vi "5785_IQ_gen_2_x_1.6GHz_max_mod_8_and_4.vi"() -> ()   [LabVIEW 2021]
uses:
  <instrlib>/_niInstr/Streaming/v1/Common/Stream State.ctl
  <vilib>/Platform/TimedLoop/XDataNode/timing_clust.ctl
  <vilib>/Platform/TimedLoop/XDataNode/nitl_modes.ctl
  <vilib>/Platform/TimedLoop/XDataNode/wakeup.ctl
  <instrlib>/FlexRIO/API/FPGA/v1/Types/Start Trigger IO Resources.ctl
  <vilib>/rvi/Emulation/niFpgaSctlEmulationGetInTimedLoop.vi
  <vilib>/rvi/Emulation/niFpgaEmulationReportErrorSimple.vi
  <vilib>/rvi/Emulation/niFpgaGetClockAttributes.vi
  <vilib>/rvi/Emulation/niFpgaCriticalErrorInLSC.vi
  7192f61d-e408-4cca-baff-cb10c33219c0.vi
  <vilib>/rvi/interface/RandomDataEmulation/nirviRandomDataMultiElementFPGAFIFO.vi
  <instcachedir>/0/nirviRandomDataMultiElementFPGAFIFO_3E9965BA1FAD4E7B8DABA31768A09B1F.lvgen/nirviRandomDataMultiElementFPGAFIFO_3E9965BA1FAD4E7B8DABA31768A09B1F_000.vi
  <vilib>/rvi/interface/RandomDataEmulation/niFpgaRandomDataHandleErrors.vi
  <instrlib>/_niInstr/DSP/v1/FPGA/Public/Sub VIs/HB Interpolator/Halfband Interpolator - IQ - 8 SPC - 2x OC.vi
  <instrlib>/_niInstr/DSP/v1/FPGA/Public/Sub VIs/Frequency Shift/Frequency Shift - 16 spc.vi
  <vilib>/rvi/eio/common/nirviEmuTemplateMethod_errors.vi
  <vilib>/Platform/TimedLoop/XDataNode/XDataNode.xnode
  <vilib>/rvi/DataTransferAndStorage/Container/XNode/niFpgaContainer.xnode
  <vilib>/rvi/interface/RandomDataEmulation/nirviRandomDataFpgaMultiElementTemplate.vi
  <vilib>/eio/EIONode/EIONode.xnode
  <vilib>/Platform/TimedLoop/XDataNode/XDNodeRunTimeDep.lvlib
  <instrlib>/_niInstr/Streaming/v1/FPGA/niInstr Streaming v1 FPGA.lvlib
  <instrlib>/FlexRIO/API/FPGA/v1/FlexRIO API FPGA v1.lvlib
  <instrlib>/FlexRIO/API/FPGA/v1/IO/NI5785/FlexRIO 5785 FPGA v1.lvlib
  <instrlib>/_niInstr/DSP/v1/FPGA/niInstr DSP v1 FPGA.lvlib
  <instrlib>/_niInstr/Basic Elements/v1/FPGA/niInstr Basic Elements v1 FPGA.lvlib
  <instrlib>/_niInstr/Streaming/v1/Common/niInstr Streaming v1 Common.lvlib
panel:
  out "pulse TX status 2":T1
  out "pulse TX status":T1
  in  "reset system clock":bool
  in  "User-defined Start Trigger - AO":bool
  in  "flexrio.trigger.start.cfg 1":u16
  out "written elements":u64
  out "IO Socket\\AO Ready For Input":bool
  in  "stream.request state 1":T2
  in  "stream.num samples 1":u64
  out "stream.metadata 1":u64
  out "stream.samples transferred 1":u64
  out "stream.state 1":T2
  out "flexrio.module.io ready 0":bool
  out "flexrio.module.io error 0":i32
  out "flexrio.module.data valid 0":bool
  # "Data Path Configuration"
  # "AI Trigger Configuration"
  # "AI Stream Configuration"
  # "AO Stream Configuration"
  # "Module Status"
  # "AO Buffer Configuration"
  # "Device Utilization\n---------------------------\nTotal Slices: 62.6% (18977 out of 30300)\nSlice Registers: 23.8% (115206 out of 484800)\nSlice LUTs: 38.2% (92532 out of 242400)\nBlock RAMs: 56.8% (341 out of 600)\nDSP48s: 0.3% (6 out of 1920)\n\nNote: Utilization numbers are for the KU040. Exact values will vary for the KU060 and KU035."
  # "User-defined Controls"
  # "AO Trigger Configuration"
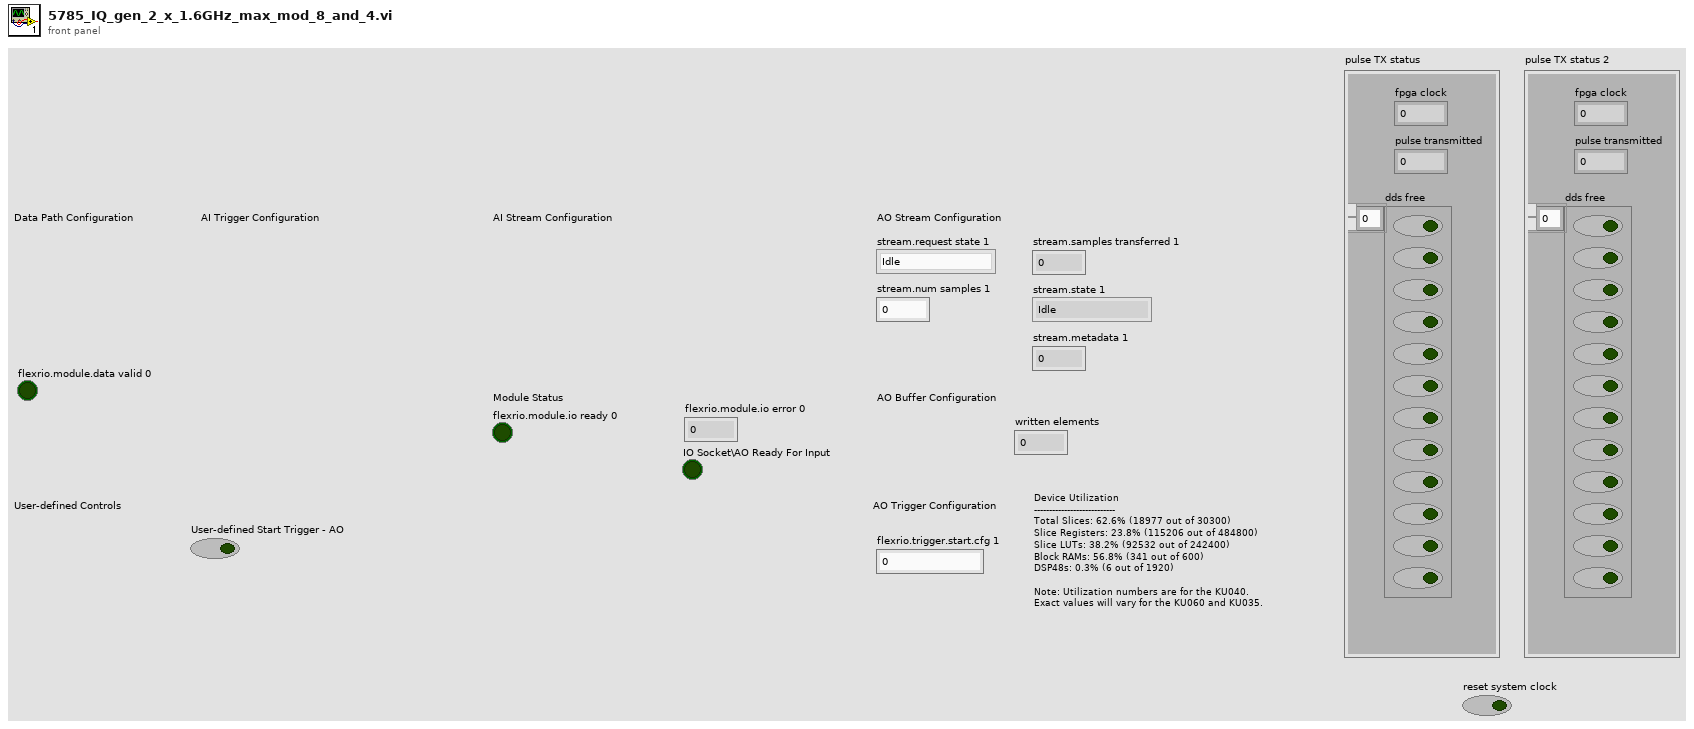
[diagram p1: front panel]
types:
  T1 = cluster{"fpga clock":u64, "pulse transmitted":u32, "dds free":bool[]}
  T2 = typedef "niInstr Streaming v1 Common.lvlib/Stream State.ctl" = enum8{"Idle", "Finite Transfer", "Continuous", "Done", "Error", "Not Ready", "Cancel"}
  T3 = typedef "XDNodeRunTimeDep.lvlib/timing_clust.ctl" = cluster{"Expected End [f-1]":u64, "Actual End [f-1]":u64, "Finished Late? [f-1]":bool, "Expected End [i-1]":u64, "Actual End [i-1]":u64, "Finished Late? [i-1]":bool, "Expected Start [i]":u64, "Actual Start [i]":u64, "Expected Start [f]":u64, "Actual Start [f]":u64, "Source Name":string, "Structure Name":string, "Period":i64, "Deadline":i64, "Offset":i64, "Start":i64, "Priority":i32, "Timeout":i32, "Mode":T4, "Wakeup Reason":T5, "Error":errorcluster, "Source Type":string, "Secondary Source Type":string, "Global End Time":u64, "Global Start Time":u64, "Frame Duration":u64, "Iteration Duration":u64, "Assigned CPU":i32, "I/O Scan Engine Mode":u32}
  T4 = typedef "XDNodeRunTimeDep.lvlib/nitl_modes.ctl" = enum32{"No Change", "Process missed periods, maintain original phase", "Discard missed periods, maintain original phase", "Process missed periods, ignore original phase", "Discard missed periods, ignore original phase"}
  T5 = typedef "XDNodeRunTimeDep.lvlib/wakeup.ctl" = enum32{"Normal", "Aborted", "Asynchronous wakeup", "Timing source error", "Timed loop error", "Timeout"}
  T6 = cluster{"Memory In":refnum<k21>, "Memory In 2":refnum<k21>, "Memory In 3":refnum<k21>, "Memory In 6":refnum<k21>, "Memory In 4":refnum<k21>, "Memory In 5":refnum<k21>, "Memory In 7":refnum<k21>, "Memory In 8":refnum<k21>}
  T7 = cluster{"clock x2":refnum<k21>, "Memory In":refnum<k21>, "Memory In 2":refnum<k21>, "Memory In 3":refnum<k21>, "Memory In 4":refnum<k21>}
  T8 = typedef "FlexRIO API FPGA v1.lvlib/Start Trigger IO Resources.ctl" = cluster{"start trigger":refnum<k21>, "started event":refnum<k21>, "start trigger for export":refnum<k21>, "start trigger for tclk":refnum<k21>}
  T9 = typedef "FlexRIO API FPGA v1.lvlib/Start Trigger Control.ctl" = cluster{"arm start":bool, "done":bool}
  T10 = typedef "niInstr DSP v1 Shared.lvlib/IQ Data.ctl" = cluster{"I":fxp<+/-,18,1>, "Q":fxp<+/-,18,1>, "overflow":bool}
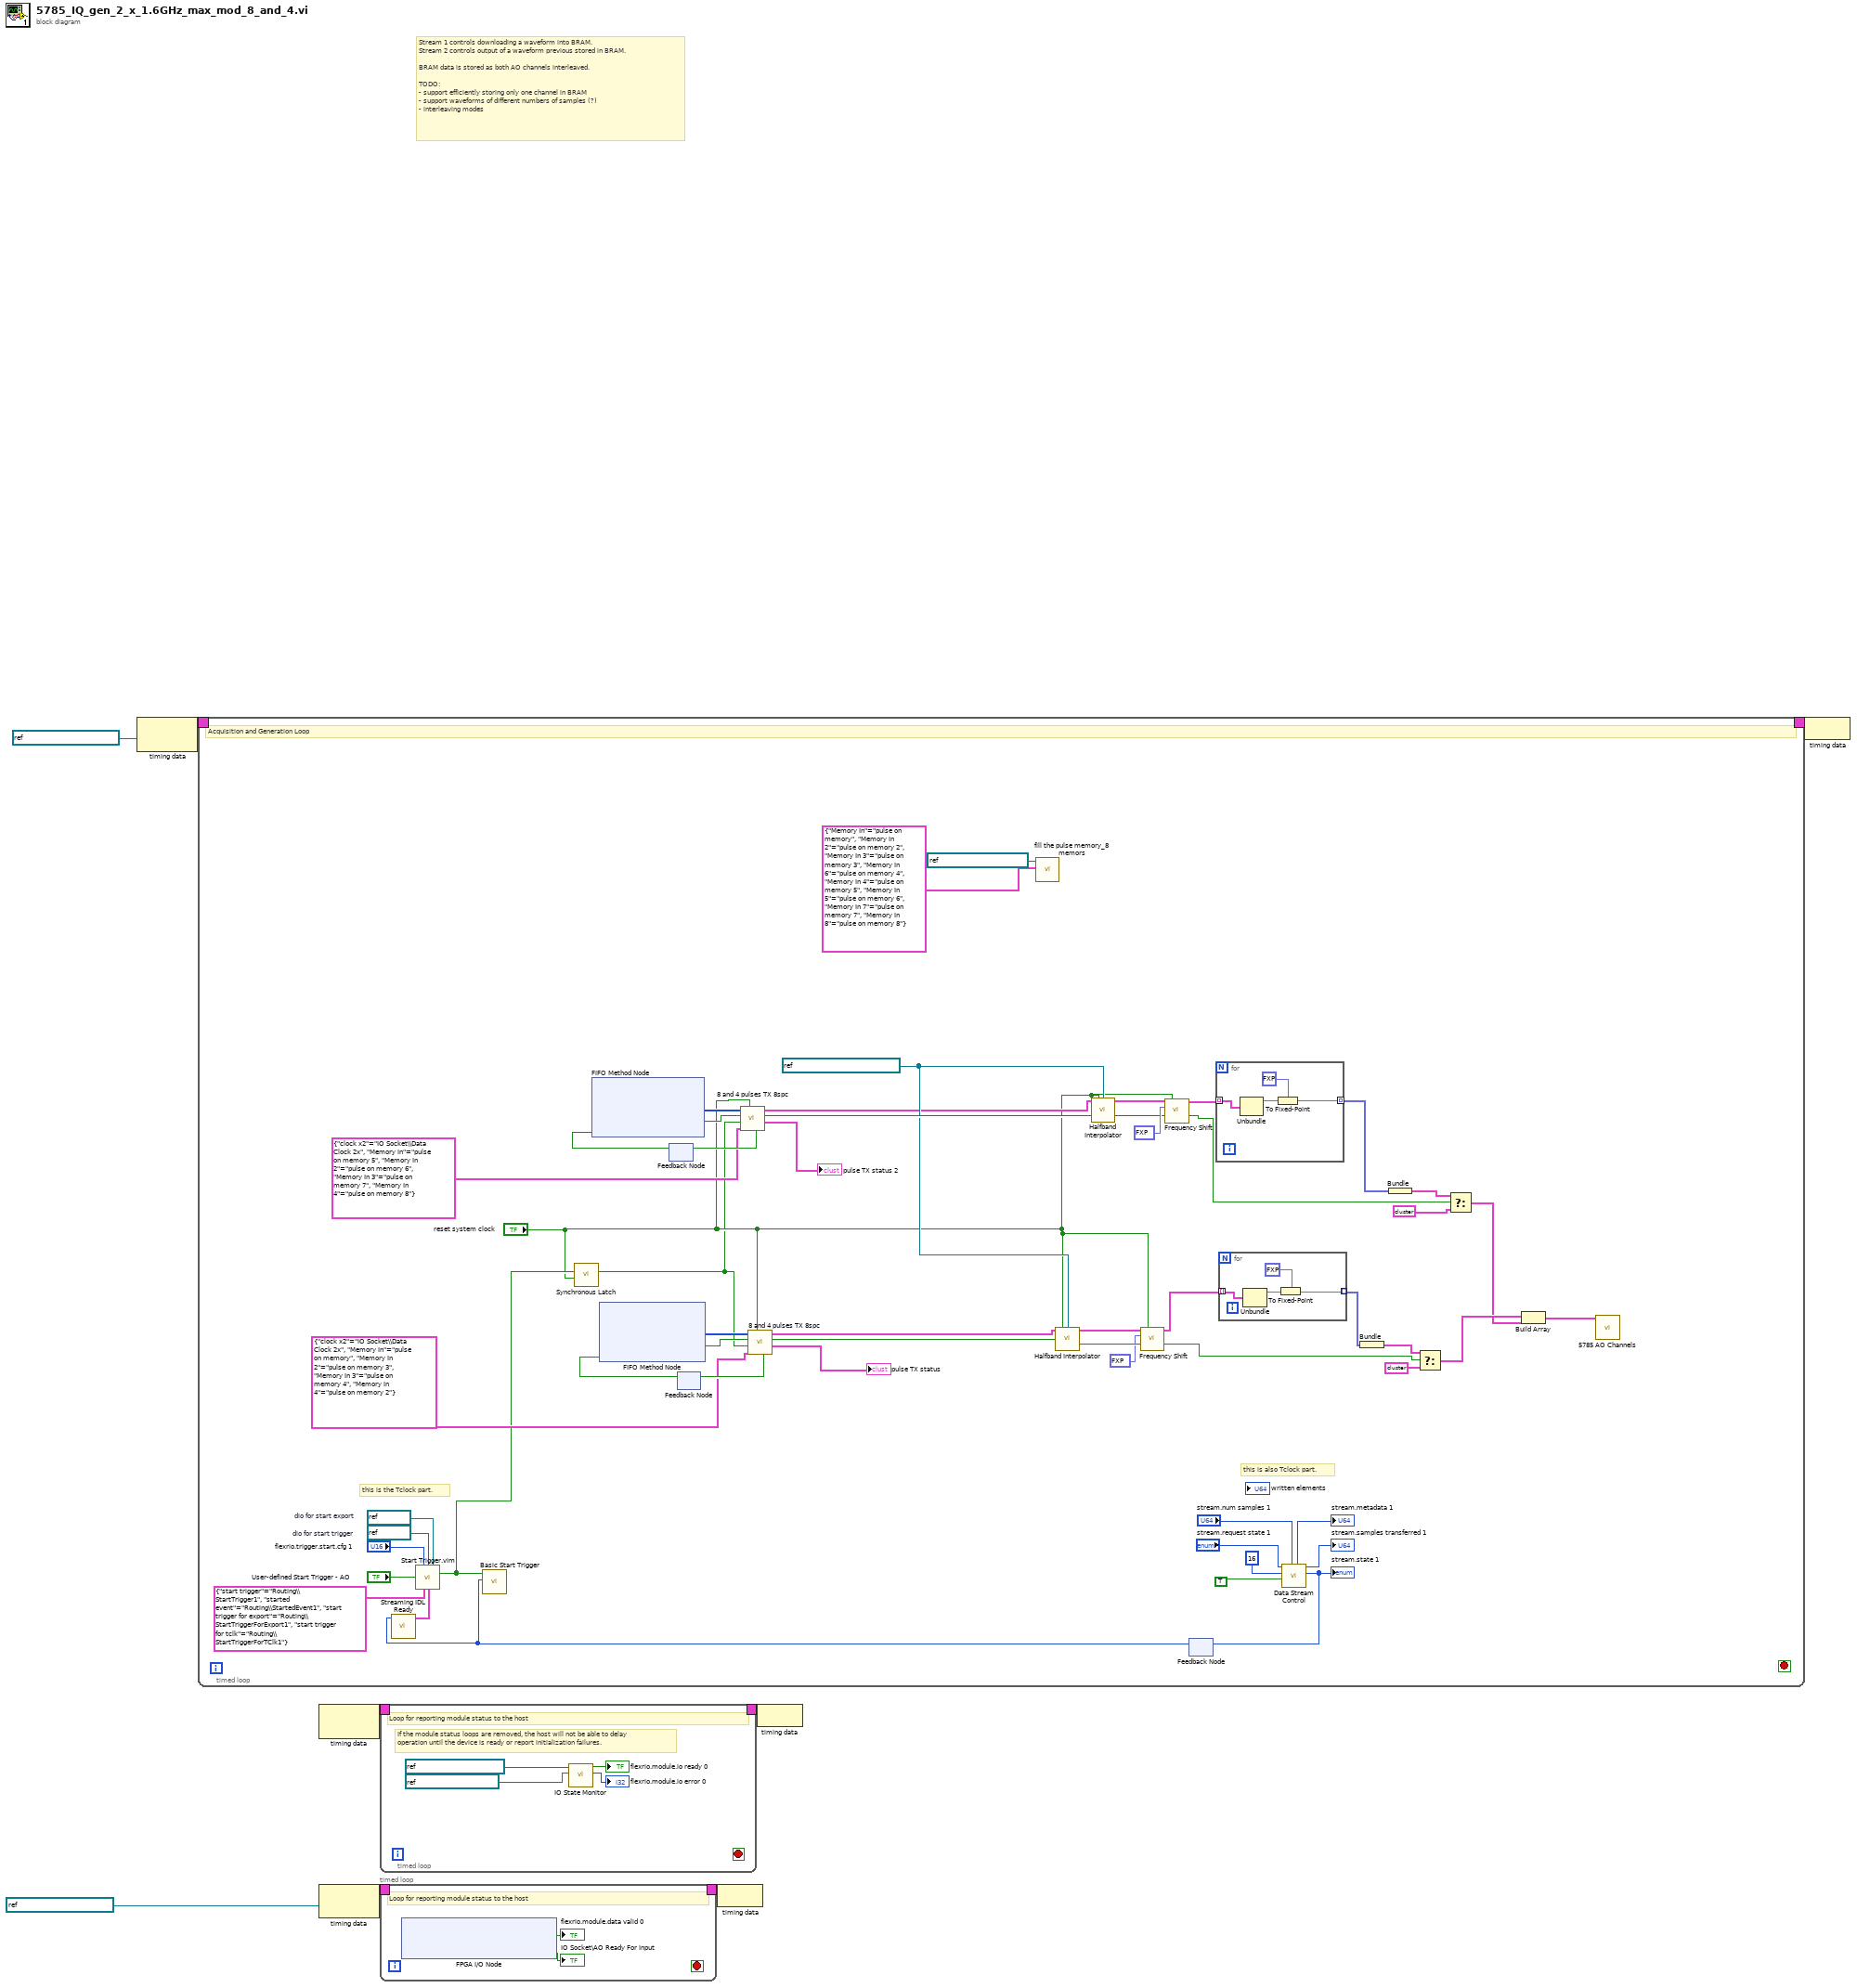
[diagram p0: block diagram]
diagram:
  # "Stream 1 controls downloading a waveform into BRAM.\nStream 2 controls output of a waveform previous stored in BRAM.\n\nBRAM data is stored as both AO channels interleaved.\n\nTODO:\n- support efficiently storing only one channel in BRAM\n- support waveforms of different numbers of samples (?)\n- interleaving modes"
  n1 = node-c288(refnum<k21> "IO Socket\\Data Clock" ("Source Name")) -> (w8:T3)
  n2 = timed-loop {
    timing: w8 -> [_]
    timing-out: [_] -> w7
    stop <- _ stop-if-true
    w40 = refnum<k21> "IO Socket\\Data Clock 2x" ("Source Name")
    w53 = refnum<k21> "DIO 2"  # dio for start trigger
    w52 = refnum<k21> "DIO 3"  # dio for start export
    # "this is also Tclock part."
    # "this is the Tclock part."
    # "Acquisition and Generation Loop"
    n3 = feedback #1() -> (w43:bool)  [unwired: 1 in]
    n4 = xnode ("FIFO Method Node")("Ready for Output"=w43) -> ("Element"=w45:u64[], "Output Valid"=w41:bool)  [unwired: 1 in, 1 out]
    n5 = feedback #2() -> (w47:bool)  [unwired: 1 in]
    n6 = xnode ("FIFO Method Node")("Ready for Output"=w47) -> ("Element"=w46:u64[], "Output Valid"=w39:bool)  [unwired: 1 in, 1 out]
    n7 = call "fill the pulse memory_8 memors.vi"("memory units"=T6 {"Memory In"="pulse on memory", "Memory In 2"="pulse on memory 2", "Memory In 3"="pulse on memory 3", "Memory In 6"="pulse on memory 4", "Memory In 4"="pulse on memory 5", "Memory In 5"="pulse on memory 6", "Memory In 7"="pulse on memory 7", "Memory In 8"="pulse on memory 8"}, "FIFO In"=refnum<k21> "fifo pulse from host") -> ()  [unwired: 10 in]
    n8 = feedback #3() -> (w50:T2)  [unwired: 1 in]
    n9 = call <instrlib>:"Streaming IDL Ready.vi"("stream.state"=w50) -> ("start trigger control"=w54:T9)  [unwired: 10 in]
    n10 = call "Start Trigger.vim"("flexrio.trigger.start.cfg 0"="flexrio.trigger.start.cfg 1", "dio start"=w53, "dio for start export"=w52, "user-defined start trigger"="User-defined Start Trigger - AO", "trigger io resources"=T8 {"start trigger"="Routing\\StartTrigger1", "started event"="Routing\\StartedEvent1", "start trigger for export"="Routing\\StartTriggerForExport1", "start trigger for tclk"="Routing\\StartTriggerForTClk1"}, "start trigger control"=w54) -> ("conditioned start trigger"=w11:bool)  [unwired: 7 in, 2 out]
    n11 = call <instrlib>:"Basic Start Trigger.vi"("stream.state"=w50, "start trigger"=w11) -> ()  [unwired: 9 in, 1 out]
    n12 = call <instrlib>:"Synchronous Latch.vi"("clear"="reset system clock", "set"=w11) -> ("out"=w9:bool)  [unwired: 9 in]
    n13 = call "8 and 4 pulses TX 8spc.vi"("reset system clock"="reset system clock", "referenses"=T7 {"clock x2"="IO Socket\\Data Clock 2x", "Memory In"="pulse on memory 5", "Memory In 2"="pulse on memory 6", "Memory In 3"="pulse on memory 7", "Memory In 4"="pulse on memory 8"}, "IQ_run"=w9, "PDW input Valid"=w41, "array PDW"=w45) -> ("pulse TX status"=→"pulse TX status 2":T1, "output valid"=w44:bool, "IQ out"=w27:T10[], "ready for input"=w42:bool)  [unwired: 3 in]
    n14 = feedback-in #1(w42) -> ()
    n15 = call "8 and 4 pulses TX 8spc.vi"("reset system clock"="reset system clock", "referenses"=T7 {"clock x2"="IO Socket\\Data Clock 2x", "Memory In"="pulse on memory", "Memory In 2"="pulse on memory 3", "Memory In 3"="pulse on memory 4", "Memory In 4"="pulse on memory 2"}, "IQ_run"=w9, "PDW input Valid"=w39, "array PDW"=w46) -> ("pulse TX status"=→"pulse TX status":T1, "output valid"=w36:bool, "IQ out"=w29:T10[], "ready for input"=w48:bool)  [unwired: 3 in]
    n16 = feedback-in #2(w48) -> ()
    n17 = call-poly <instrlib>:"Halfband Interpolator.vi"("data in"=w29, "reset"="reset system clock", "clock x 2"=w40, "input valid"=w36) -> ("data out"=w20:T10[], "output valid"=w21:bool)  [unwired: 8 in, 2 out]
    n18 = call-poly <instrlib>:"Halfband Interpolator.vi"("data in"=w27, "reset"="reset system clock", "clock x 2"=w40, "input valid"=w44) -> ("data out"=w14:T10[], "output valid"=w15:bool)  [unwired: 8 in, 2 out]
    n19 = call-poly <instrlib>:"Frequency Shift.vi"("data in"=w20, "reset"="reset system clock", "frequency shift"=fxp<+/-,48,0> 0.25, "input valid"=w21) -> ("data out"=w18:T10[], "output valid"=w19:bool)  [unwired: 8 in, 2 out]
    n20 = call-poly <instrlib>:"Frequency Shift.vi"("data in"=w14, "reset"="reset system clock", "frequency shift"=fxp<+/-,48,0> 0.25, "input valid"=w15) -> ("data out"=w13:T10[], "output valid"=w12:bool)  [unwired: 8 in, 2 out]
    n21 = for {
      tunnel: w13 -> [w67] mode=indexing
      tunnel: [w64] -> w37 mode=indexing
      n22 = Unbundle(w67) -> ("I"=w66:fxp<+/-,18,1>)  [unwired: 2 out]
      n23 = To Fixed-Point(fixed-point type=fxp<+/-,12,1> 0.0 ("element"), number=w66) -> (fixed-point=w64:fxp<+/-,12,1>)
    }
    n24 = for {
      tunnel: w18 -> [w71] mode=indexing
      tunnel: [w68] -> w38 mode=indexing
      n25 = Unbundle(w71) -> ("I"=w70:fxp<+/-,18,1>)  [unwired: 2 out]
      n26 = To Fixed-Point(fixed-point type=fxp<+/-,12,1> 0.0 ("element"), number=w70) -> (fixed-point=w68:fxp<+/-,12,1>)
    }
    n27 = call <instrlib>:"Data Stream Control.vi"("stream.num samples 0"="stream.num samples 1", "data valid"=TRUE, "element count"=u16 16, "stream.request state 0"="stream.request state 1") -> ("stream.state 0"=w56:T2, "stream.samples transferred 0"=→"stream.samples transferred 1":u64, "stream.metadata 0"=→"stream.metadata 1":u64)  [unwired: 3 in, 2 out]
    "stream.state 1" <- w56
    n28 = feedback-in #3(w56) -> ()
    n29 = Bundle(w38) -> (w35:cluster{fxp<+/-,12,1>[]})  [unwired: 1 in]
    n30 = Bundle(w37) -> (w31:cluster{fxp<+/-,12,1>[]})  [unwired: 1 in]
    n31 = Select(t=w35, s=w19, f=cluster{fxp<+/-,12,1>[]} {[0.0, 0.0, 0.0, 0.0, 0.0, 0.0, 0.0, 0.0, 0.0, 0.0, 0.0, 0.0, 0.0, 0.0, 0.0, 0.0]}) -> (s? t:f=w34:cluster{fxp<+/-,12,1>[]})
    n32 = Select(t=w31, s=w12, f=cluster{fxp<+/-,12,1>[]} {[0.0, 0.0, 0.0, 0.0, 0.0, 0.0, 0.0, 0.0, 0.0, 0.0, 0.0, 0.0, 0.0, 0.0, 0.0, 0.0]}) -> (s? t:f=w30:cluster{fxp<+/-,12,1>[]})
    n33 = Build Array(w34, w30) -> (w61:cluster{fxp<+/-,12,1>[]}[])
    n34 = call <instrlib>:"5785 AO Channels.vi"("all channels"=w61) -> ()  [unwired: 15 in]
  }
  n35 = node-c288() -> (w5:T3)  [unwired: 1 in]
  n36 = node-c288(refnum<k21> "IO Socket\\Data Clock" ("Source Name")) -> (w3:T3)
  n37 = timed-loop {
    timing: w5 -> [_]
    timing-out: [_] -> w4
    stop <- _ stop-if-true
    # "If the module status loops are removed, the host will not be able to delay operation until the device is ready or report initialization failures."
    # "Loop for reporting module status to the host"
    n38 = call <instrlib>:"IO State Monitor.vi"("io error resource"=refnum<k21> "IO Socket\\IO Error" ("FPGA I/O In"), "io ready resource"=refnum<k21> "IO Socket\\IO Ready" ("FPGA I/O In")) -> ("flexrio.module.io error 0"=→"flexrio.module.io error 0":i32, "flexrio.module.io ready 0"=→"flexrio.module.io ready 0":bool)  [unwired: 8 in]
  }
  n39 = timed-loop {
    timing: w3 -> [_]
    timing-out: [_] -> w2
    stop <- _ stop-if-true
    # "Loop for reporting module status to the host"
    n40 = xnode "FPGA I/O Node"() -> ("IO Socket\\AI Data Valid"=→"flexrio.module.data valid 0":bool, "IO Socket\\AO Ready For Input"=→"IO Socket\\AO Ready For Input":bool)  [unwired: 2 in, 2 out]
  }
  n41 = node-c288(w2) -> ()
  n42 = node-c288(w4) -> ()
  n43 = node-c288(w7) -> ()
